vi "EOL CAN_Get_Motor_Software_Level.vi"(11 "NetworkObjHandle":T1) -> (1 "Customer Part Number":string, 2 "SW Level":string, 3 "Response Good?":bool, 5 "TxRx Data":string[][](array[string]))   [LabVIEW 2018]
uses:
  <vilib>/nican/nican.llb/xobjhandle.ctl
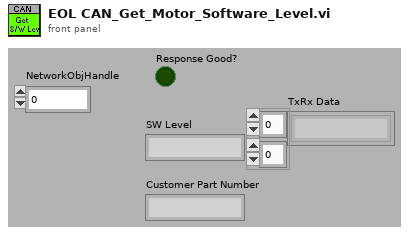
[diagram p1: front panel]
types:
  T1 = typedef "xobjhandle.ctl" = u32
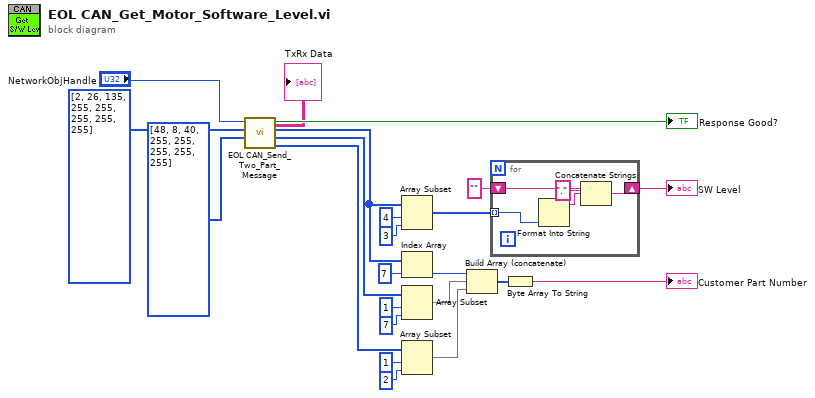
[diagram p0: block diagram]
diagram:
  n1 = call <userlib>:"EOL CAN_Send_Two_Part_Message.vi"("Tx 2"=u8[] [48, 8, 40, 255, 255, 255, 255, 255] ("Transmit Data"), "Tx 1"=u8[] [2, 26, 135, 255, 255, 255, 255, 255] ("Transmit Data"), "NetworkObjHandle"="NetworkObjHandle") -> ("Array 23"=w4:u8[], "Array 22"=w3:u8[], "Array 21"=w2:u8[], "Response Good?"=→"Response Good?":bool, "TxRx Data"=→"TxRx Data":string[][])  [unwired: 4 in]
  n2 = Array Subset(array=w2, index=4, length=3) -> (w17:u8[])
  n3 = Index Array(array=w2, index=7) -> (element=w12:u8)
  n4 = Array Subset(array=w3, index=1, length=7) -> (w13:u8[])
  n5 = Array Subset(array=w4, index=1, length=2) -> (w14:u8[])
  n6 = Build Array (concatenate)(w12, w13, w14) -> (w16:u8[])
  n7 = for {
    tunnel: w17 -> [w28] mode=indexing
    shift-right: [w26] -> w19
    shift-left: "" -> [w25]
    n8 = Format Into String(w28) -> (resulting string=w27:string)  [unwired: 3 in, 1 out]
    n9 = Concatenate Strings(w25, w27, "." ("string")) -> (w26:string)
  }
  "SW Level" <- w19
  n10 = Byte Array To String(unsigned byte array=w16) -> (string=→"Customer Part Number":string)
